vi "checkLBValueNoEvent.vi"() -> (0 "light barriers":bool[](array[boolean]))   [LabVIEW 2012]
uses:
  GlobalArduino.vi
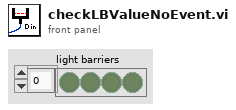
[diagram p1: front panel]
types:
  T1 = typedef "Semaphore RefNum" = refnum<k1>
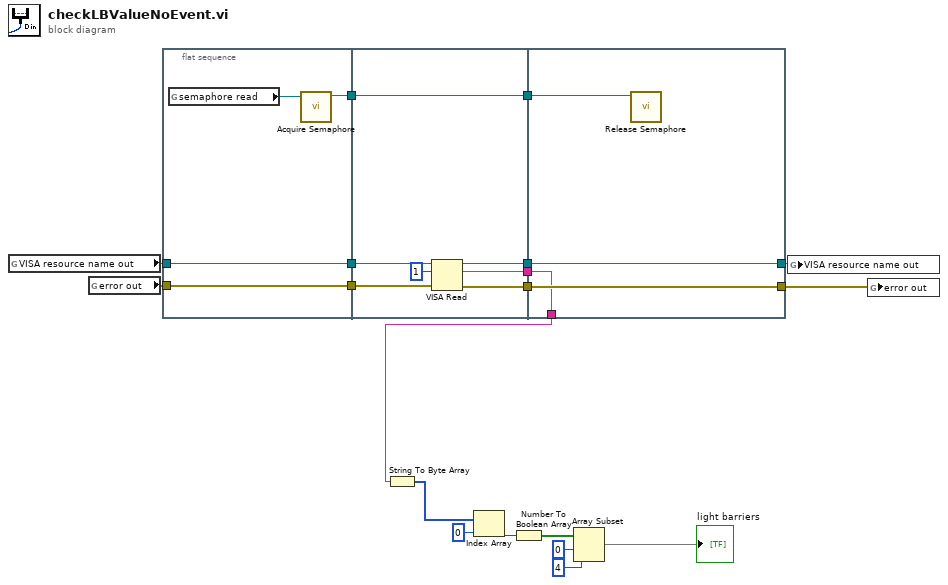
[diagram p0: block diagram]
diagram:
  n1 = global read "GlobalArduino.vi" "VISA resource name out"() -> (w12:refnum<visa-resource-name>)
  n2 = global read "GlobalArduino.vi" "error out"() -> (w11:errorcluster)
  n3 = flat-sequence {
    tunnel: w11 -> [w22]
    tunnel: w12 -> [w23]
    tunnel: [w23] -> w8
    tunnel: [w22] -> w7
    tunnel: [w20] -> w1
    tunnel: w8 -> [w29]
    tunnel: w7 -> [w28]
    tunnel: [w27] -> w6
    tunnel: [w26] -> w5
    tunnel: [w25] -> w4
    tunnel: [w24] -> w2
    tunnel: w1 -> [w24]
    tunnel: [w33] -> w9
    tunnel: [w34] -> w10
    tunnel: w6 -> [w34]
    tunnel: w5 -> [w33]
    tunnel: w4 -> [w32]
    tunnel: [w32] -> w3
    tunnel: w2 -> [w31]
    frame #0 {
      n4 = global read "GlobalArduino.vi" "semaphore read"() -> (w21:T1)
      n5 = call <vilib>:"Acquire Semaphore.vi"("semaphore"=w21) -> ("semaphore out"=w20:T1)  [unwired: 4 in, 2 out]
    }
    frame #1 {
      n6 = VISA Read(VISA resource name=w29, byte count=u32 1, error in (no error)=w28) -> (VISA resource name out=w27:refnum<visa-resource-name>, read buffer=w25:string, error out=w26:errorcluster)  [unwired: 1 out]
    }
    frame #2 {
      n7 = call <vilib>:"Release Semaphore.vi"("semaphore"=w31) -> ()  [unwired: 5 in, 2 out]
    }
  }
  n8 = String To Byte Array(string=w3) -> (unsigned byte array=w19:u8[])
  n9 = Index Array(array=w19, index=0) -> (element=w17:u8)
  n10 = Number To Boolean Array(number=w17) -> (Boolean array=w16:bool[])
  n11 = Array Subset(array=w16, index=0, length=4) -> (→"light barriers":bool[])
  n12 = global write "GlobalArduino.vi" "VISA resource name out"(w10) -> ()
  n13 = global write "GlobalArduino.vi" "error out"(w9) -> ()
